vi "DDE Master Control.vi"(5 "timeout(-1)":i32=-1, 9 "input":T2={"trans type"=1, "refnums"=[], "data1"="excel", "data2"="sheet1", "status"=FALSE} {"refnums" format="%.0x"}) -> (0 "error out":errorcluster, 1 "changed?":bool, 2 "data":string, 3 "refnum":u32 format="%.0x", 4 "changed values":T1(array[cluster]))   [LabVIEW 2014]
panel:
  in  "datatype":T1(array[cluster])
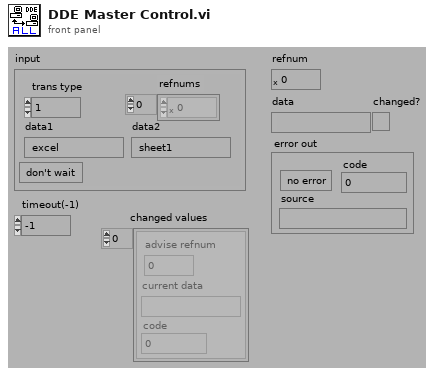
[diagram p1: front panel]
types:
  T1 = cluster{"advise refnum":u32, "current data":string, "code":i32}[]
  T2 = cluster{"trans type":i8, "refnums":u32[], "data1":string, "data2":string, "status":bool}
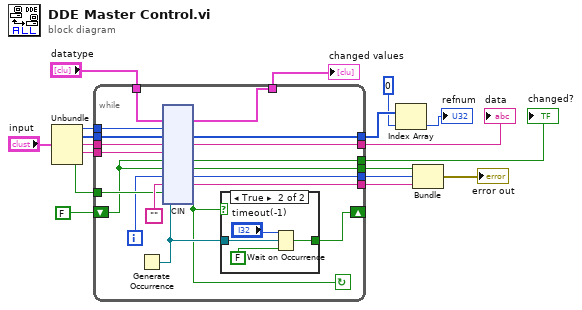
[diagram p0: block diagram]
diagram:
  n1 = Unbundle("input") -> ("trans type"=w12:i8, "refnums"=w9:u32[], "data1"=w17:string, "data2"=w15:string, "status"=w8:bool)
  n2 = while {
    tunnel: "datatype" -> [w19]
    tunnel: [w20] -> w2
    tunnel: [w22] -> w6
    shift-left: FALSE -> [w21]
    shift-right: [w24] -> _
    tunnel: w8 -> [w25]
    tunnel: [w27] -> w4
    tunnel: w9 -> [w28]
    tunnel: [w34] -> w14
    tunnel: [w35] -> w13
    tunnel: w15 -> [w31]
    tunnel: w17 -> [w36]
    tunnel: [w33] -> w16
    tunnel: [w37] -> w10
    tunnel: w12 -> [w30]
    i -> [w23]
    stop <- w26 continue-if-true
    n3 = Generate Occurrence() -> (w29:refnum<k4>)
    n4 = cin(w19, w30, w28, w36, w31, w21, w21, w23, "", w25, w29) -> (w20:T1, w27:u32[], w35:string, w22:bool, w34:bool, w33:i32, w37:string, w26:bool)  [unwired: 3 in]
    n5 = case shown="True" w26 {
      selector: w26 -> [w38 _]
      tunnel: w29 -> [_ w42]
      tunnel: [w38 w39] -> w24
      frame False {
      }
      frame True {
        n6 = Wait on Occurrence(1:FALSE, 2:w42, 3:"timeout(-1)") -> (0:w39:bool)
      }
    }
  }
  "data" <- w13
  "changed?" <- w6
  "changed values" <- w2
  n7 = Index Array(array=w4, index=0) -> (element=→"refnum":u32)
  n8 = Bundle(w14, w16, w10) -> (→"error out":errorcluster)  [unwired: 1 in]
